vi "KeDSO Try Fetch Data.vi"(8 "error in":errorcluster, 11 "keysight dso":T3 {"bw limit [Hz]" format="%#_6p"; "channels"."Offset [V]" min=0.0 format="%#_6p"; "channels"."Range [Vpk]" min=0.0 format="%#_6p"; "channels"."Channel" min=1}) -> (0 "error out":errorcluster, 1 "aux data":T2, 2 "sample data":T1, 3 "keysight dso out":T3 {"bw limit [Hz]" format="%#_6p"; "channels"."Offset [V]" min=0.0 format="%#_6p"; "channels"."Range [Vpk]" min=0.0 format="%#_6p"; "channels"."Channel" min=1}, 4 "fetching done?":bool)   [LabVIEW 2020]
doc: "This is called after KeDSO Initiate Digitizing Process.vi repetitively until it returns sample data. It is non-blocking VI."
uses:
  KeDSO session.ctl
  KeDSO Virtual Channel.ctl
  KeDSO Trigger Setup.ctl
  KeDSO Trigger Source.ctl
  KeDSO Record Aux Data.ctl
  KeDSO Record Sample Data.ctl
  Agilent 90000 Series.lvlib
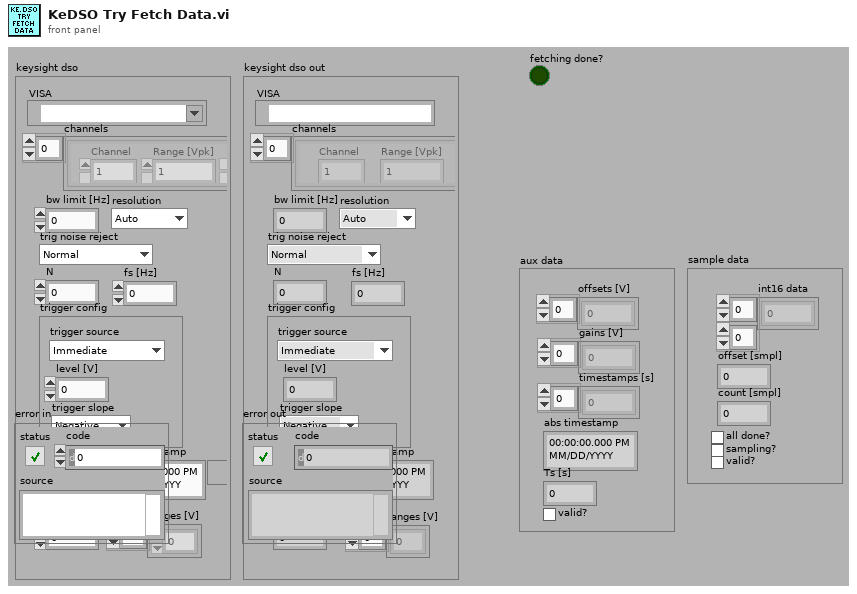
[diagram p1: front panel]
types:
  T1 = typedef "KeDSO Record Sample Data.ctl" = cluster{"int16 data":i16[][], "offset [smpl]":i64, "count [smpl]":i64, "all done?":bool, "sampling?":bool, "valid?":bool}
  T2 = typedef "KeDSO Record Aux Data.ctl" = cluster{"offsets [V]":dbl[], "gains [V]":dbl[], "timestamps [s]":dbl[], "abs timestamp":timestamp, "Ts [s]":dbl, "valid?":bool}
  T3 = typedef "KeDSO session.ctl" = cluster{"VISA":refnum<visa-resource-name>, "channels":T4[], "bw limit [Hz]":dbl, "resolution":enum16{"Auto", "Bits 9", "Bits 10", "Bits 11", "Bits 12"}, "trig noise reject":enum16{"Normal", "High Sensitivity"}, "N":i64, "trigger config":T5, "fs [Hz]":dbl, "timeout stop":timestamp, "waiting for opc":bool, "fetch offset [smpl]":i64, "abs timestamp":timestamp, "ranges [V]":dbl[]}
  T4 = typedef "KeDSO Virtual Channel.ctl" = cluster{"Channel":i32, "Range [Vpk]":dbl, "btn clr":bool, "btn up":bool, "btn down":bool, "Offset [V]":dbl, "Coupling":enum16{"DC", "DC50", "AC", "LFR1"}, "bw limit enab":bool}
  T5 = typedef "KeDSO Trigger Setup.ctl" = cluster{"trigger source":T6, "level [V]":dbl, "trigger slope":enum16{"Negative", "Positive", "Either"}}
  T6 = typedef "KeDSO Trigger Source.ctl" = enum16{"Immediate", "Level", "AUX"}
  T7 = cluster{"Actual Samples":i32, "Absolute Initial X":dbl, "Relative Initial X":dbl, "X Increment":dbl, "Offset":dbl, "Gain":dbl, "Reserved1":dbl, "Reserved2":dbl}
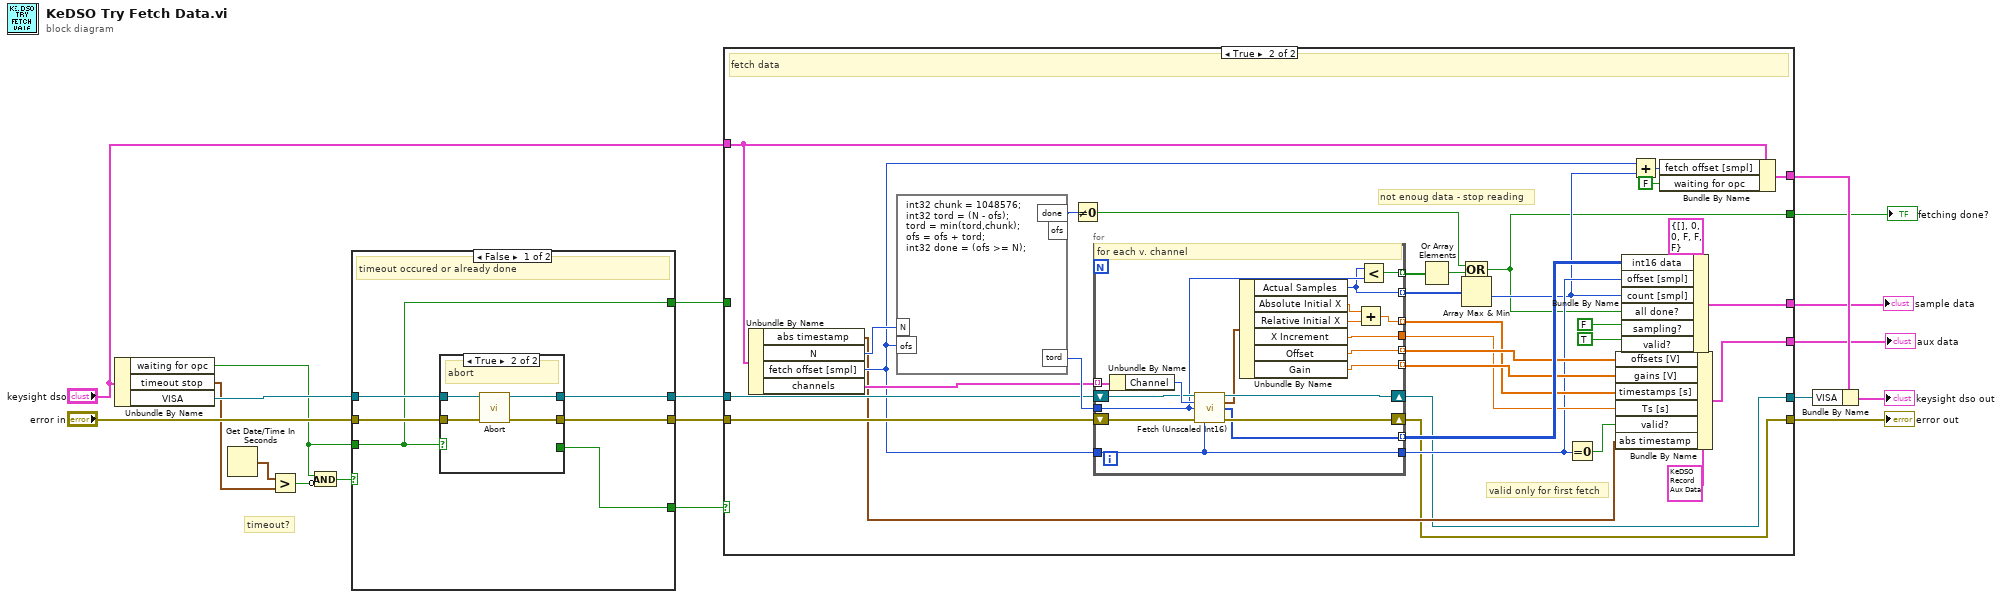
[diagram p0: block diagram]
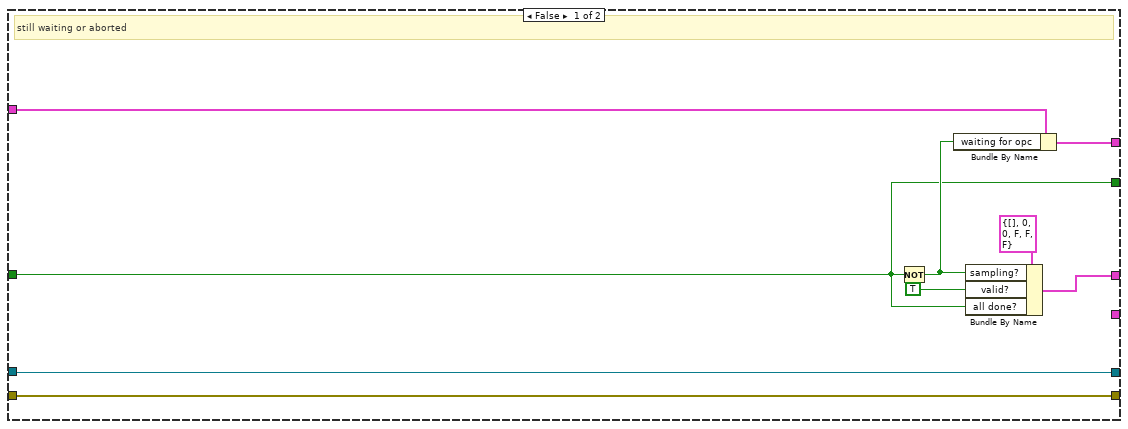
[diagram p2: hidden frame]
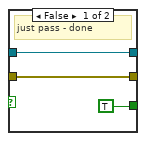
[diagram p3: hidden frame]
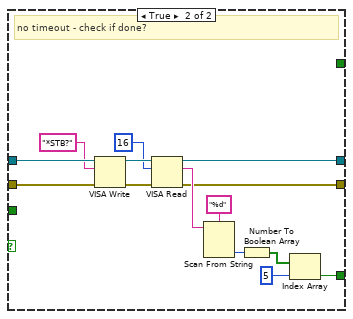
[diagram p4: hidden frame]
diagram:
  # "timeout?"
  n1 = Unbundle By Name("keysight dso") -> ("waiting for opc"=w12:bool, "timeout stop"=w16:timestamp, "VISA"=w17:refnum<visa-resource-name>)
  n2 = Get Date/Time In Seconds() -> (seconds since 1Jan1904=w15:timestamp)
  n3 = Greater?(x=w15, y=w16) -> (0:w13:bool)
  n4 = Compound Arithmetic op=AND(w12, invert w13) -> (w14:bool)
  n5 = case shown="False" w14 {
    tunnel: "error in" -> [w25 w46]
    tunnel: w17 -> [w24 w45]
    tunnel: [w22 w35] -> w10
    tunnel: [w23 w34] -> w9
    tunnel: w12 -> [w20 _]
    tunnel: [w21 w33] -> w11
    tunnel: [w20 _] -> w2
    frame False {
      # "timeout occured or already done"
      n6 = case shown="True" w20 {
        tunnel: w25 -> [w28 w32]
        tunnel: w24 -> [w27 w31]
        tunnel: [w27 w30] -> w23
        tunnel: [w28 w29] -> w22
        tunnel: [TRUE _] -> w21
        frame False {
          # "just pass - done"
        }
        frame True {
          # "abort"
          n7 = call "Abort.vi"("error in (no error)"=w32, "VISA resource name"=w31) -> ("error out"=w29:errorcluster, "VISA resource name out"=w30:refnum<visa-resource-name>)  [unwired: 8 in]
        }
      }
    }
    frame True {
      # "no timeout - check if done?"
      n8 = VISA Write(VISA resource name=w45, write buffer="*STB?", error in (no error)=w46) -> (VISA resource name out=w43:refnum<visa-resource-name>, error out=w42:errorcluster)  [unwired: 1 out]
      n9 = VISA Read(VISA resource name=w43, byte count=u32 16, error in (no error)=w42) -> (VISA resource name out=w34:refnum<visa-resource-name>, read buffer=w40:string, error out=w35:errorcluster)  [unwired: 1 out]
      n10 = Scan From String(format string="%d", input string=w40) -> (output 1=w38:i32)  [unwired: 3 in, 3 out]
      n11 = Number To Boolean Array(number=w38) -> (Boolean array=w37:bool[])
      n12 = Index Array(array=w37, index=5) -> (element=w33:bool)
    }
  }
  n13 = case shown="True" w11 {
    tunnel: w10 -> [w48 w88]
    tunnel: w9 -> [w49 w84]
    tunnel: "keysight dso" -> [w51 w67]
    tunnel: [w55 w62] -> w7
    tunnel: [w48 w58] -> w6
    tunnel: [w49 w57] -> w5
    tunnel: [w54 w61] -> w4
    tunnel: [_ w60] -> w3
    tunnel: w2 -> [w47 _]
    tunnel: [w47 w56] -> w1
    frame False {
      # "still waiting or aborted"
      n14 = Not(x=w47) -> (.not. x?=w50:bool)
      n15 = Bundle By Name(cluster=w51, "waiting for opc"=w50) -> (w55:T3)
      n16 = Bundle By Name(cluster=T1 {"int16 data"=[], "offset [smpl]"=0, "count [smpl]"=0, "all done?"=FALSE, "sampling?"=FALSE, "valid?"=FALSE} ("sample data"), "sampling?"=w50, "valid?"=TRUE, "all done?"=w47) -> (w54:T1)
    }
    frame True {
      # "valid only for first fetch"
      # "not enoug data - stop reading"
      # "fetch data"
      n17 = Unbundle By Name(w67) -> ("abs timestamp"=w59:timestamp, "N"=w87:i64, "fetch offset [smpl]"=w65:i64, "channels"=w85:T4[])
      n18 = formula code="int32 chunk = 1048576;\nint32 tord = (N - ofs);\ntord = min(tord,chunk);\nofs = ofs + tord;\nint32 done = (ofs >= N);"("N"=w87, "ofs"=w65) -> ("tord"=w86:i32, "done"=w81:i32)  [unwired: 1 out]
      n19 = Not Equal To 0?(x=w81) -> (x != 0?=w80:bool)
      n20 = for {
        tunnel: w65 -> [w92]
        tunnel: w86 -> [w98]
        tunnel: w85 -> [w105] mode=indexing
        shift-right: [w102] -> w57
        shift-left: w84 -> [w103]
        shift-right: [w101] -> w58
        shift-left: w88 -> [w106]
        tunnel: [w99] -> w77 mode=indexing
        tunnel: [w97] -> w83 mode=indexing
        tunnel: [w96] -> w79 mode=indexing
        tunnel: [w95] -> w73 mode=indexing
        tunnel: [w94] -> w72 mode=indexing
        tunnel: [w89] -> w71 mode=indexing
        tunnel: [w93] -> w70
        tunnel: [w92] -> w68
        # "for each v. channel"
        n21 = Unbundle By Name(w105) -> ("Channel"=w104:i32)
        n22 = call "Fetch (Unscaled Int16).vi"("VISA resource name"=w103, "Measurement Source (1: Channel 1)"=w104, "Number of Samples (1000)"=w98, "error in (no error)"=w106, "Offset (0)"=w92) -> ("VISA resource name out"=w102:refnum<visa-resource-name>, "Waveform Information"=w100:T7, "Waveform Data"=w99:i16[], "error out"=w101:errorcluster)  [unwired: 7 in]
        n23 = Unbundle By Name(w100) -> ("Actual Samples"=w96:i32, "Absolute Initial X"=w91:dbl, "Relative Initial X"=w90:dbl, "X Increment"=w93:dbl, "Offset"=w95:dbl, "Gain"=w94:dbl)
        n24 = Add(x=w91, y=w90) -> (x+y=w89:dbl)
        n25 = Less?(x=w96, y=w98) -> (x < y?=w97:bool)
      }
      n26 = Or Array Elements(Boolean array=w83) -> (logical OR=w82:bool)
      n27 = Array Max & Min(array=w79) -> (min value=w64:i32)  [unwired: 3 out]
      n28 = Compound Arithmetic op=OR(w80, w82) -> (w56:bool)
      n29 = Equal To 0?(x=w68) -> (x = 0?=w69:bool)
      n30 = Bundle By Name(cluster=T2 {"offsets [V]"=[], "gains [V]"=[], "timestamps [s]"=[], "abs timestamp"=timestamp(0 s since 1904-01-01), "Ts [s]"=0.0, "valid?"=FALSE} ("aux data"), "offsets [V]"=w73, "gains [V]"=w72, "timestamps [s]"=w71, "Ts [s]"=w70, "valid?"=w69, "abs timestamp"=w59) -> (w60:T2)
      n31 = Bundle By Name(cluster=T1 {"int16 data"=[], "offset [smpl]"=0, "count [smpl]"=0, "all done?"=FALSE, "sampling?"=FALSE, "valid?"=FALSE} ("sample data"), "int16 data"=w77, "offset [smpl]"=w68, "count [smpl]"=w64, "all done?"=w56, "sampling?"=FALSE, "valid?"=TRUE) -> (w61:T1)
      n32 = Add(x=w65, y=w64) -> (x+y=w66:i64)
      n33 = Bundle By Name(cluster=w67, "fetch offset [smpl]"=w66, "waiting for opc"=FALSE) -> (w62:T3)
    }
  }
  "error out" <- w6
  "aux data" <- w3
  "sample data" <- w4
  "fetching done?" <- w1
  n34 = Bundle By Name(cluster=w7, "VISA"=w5) -> (→"keysight dso out":T3)
